vi "updateWaypoints.vi"(8 "error in (no error)":errorcluster, 11 "RoundBuoys in":refnum<class "RoundBuoy.lvclass">) -> (0 "error out":errorcluster, 3 "RoundBuoys out":refnum<class "RoundBuoy.lvclass">)   [LabVIEW 2011, in "RoundBuoy.lvclass"]
uses:
  RoundBuoy.lvclass
  2 Globals/2 Global.vi
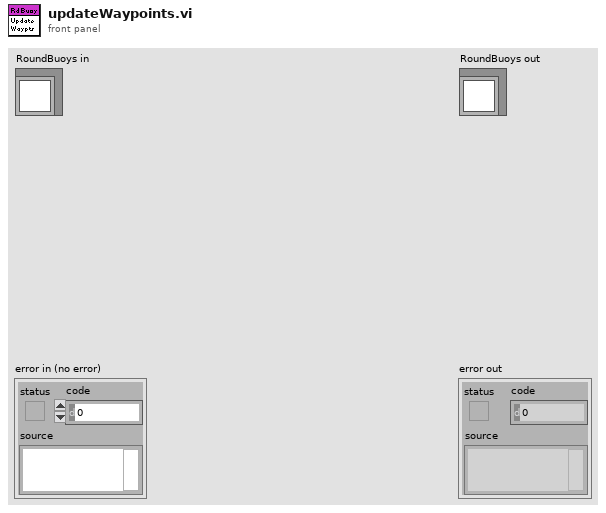
[diagram p1: front panel]
types:
  T1 = typedef "Waypoints List.ctl" = refnum<class "Waypoint.lvclass">[]
  T2 = typedef "Current Waypoint.ctl" = i32
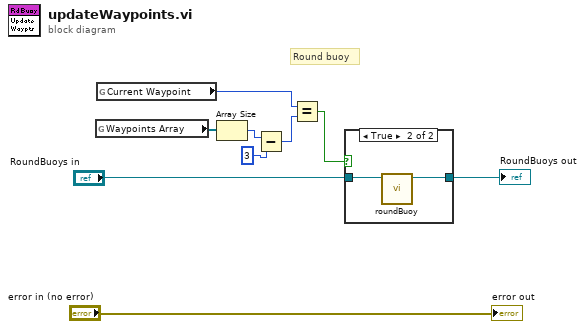
[diagram p0: block diagram]
diagram:
  # "Round buoy"
  n1 = global read "2 Global.vi" "Waypoints Array"() -> (w8:T1)
  n2 = global read "2 Global.vi" "Current Waypoint"() -> (w6:T2)
  n3 = Array Size(array=w8) -> (size(s)=w7:i32)
  n4 = Subtract(x=w7, y=3) -> (x-y=w5:i32)
  n5 = Equal?(x=w6, y=w5) -> (x = y?=w4:bool)
  n6 = case shown="True" w4 {
    tunnel: "RoundBuoys in" -> [w10 w12]
    tunnel: [w10 w11] -> w2
    frame False {
    }
    frame True {
      n7 = call "roundBuoy.vi"("RoundBuoys in"=w12) -> ("RoundBuoys out"=w11:refnum<class "RoundBuoy.lvclass">)  [unwired: 10 in]
    }
  }
  "RoundBuoys out" <- w2
  "error out" <- "error in (no error)"
